vi "Add Tx UDP Section and Status Channels.vi"(8 "error in":errorcluster, 10 "Tx UDP configuration":T7(array[cluster]) {"sapPorts"."Parameters"."Parameter"."encoding" items=["BNR", "BCD", "Discrete"]; "commPorts"."Parameters"."Parameter"."encoding" items=["BNR", "BCD", "Discrete"]; "tx_udp_setup"."NumOfSubVl" format="%.0b"; "tx_udp_setup"."NetSelect" items=["FDX_TX_FRAME_DLY_A", "FDX_TX_FRAME_DLY_B", "FDX_TX_FRAME_BOTH", "FDX_TX_FRAME_ONLY_A", "FDX_TX_FRAME_ONLY_B"]}, 11 "port ref":T8 format="%.0x") -> (0 "error out":errorcluster, 3 "port ref out":T8 format="%.0x")   [LabVIEW 2020, in "AIM ARINC 664 Scripting.lvlib"]
doc: "Add a TX UDP page and status pages based on the Tx UDP configuration."
uses:
  AIM ARINC 664 Scripting.lvlib
  <vilib>/NI VeriStand/Custom Device API/Custom Device Item Ref.ctl
  <vilib>/NI VeriStand/Custom Device API/Custom Device API.lvlib
  Import/_typedefs/frame_parameter_definition.ctl
  Import/AIM ARINC 664 Import.lvlib
  Import/_typedefs/tx_udp_setup.ctl
  Import/_typedefs/frame_parameter.ctl
  Import/_typedefs/port_tx_udp_comm.ctl
  Import/_typedefs/port_tx_udp_sap.ctl
  Shared/Encoding (Arinc664).ctl
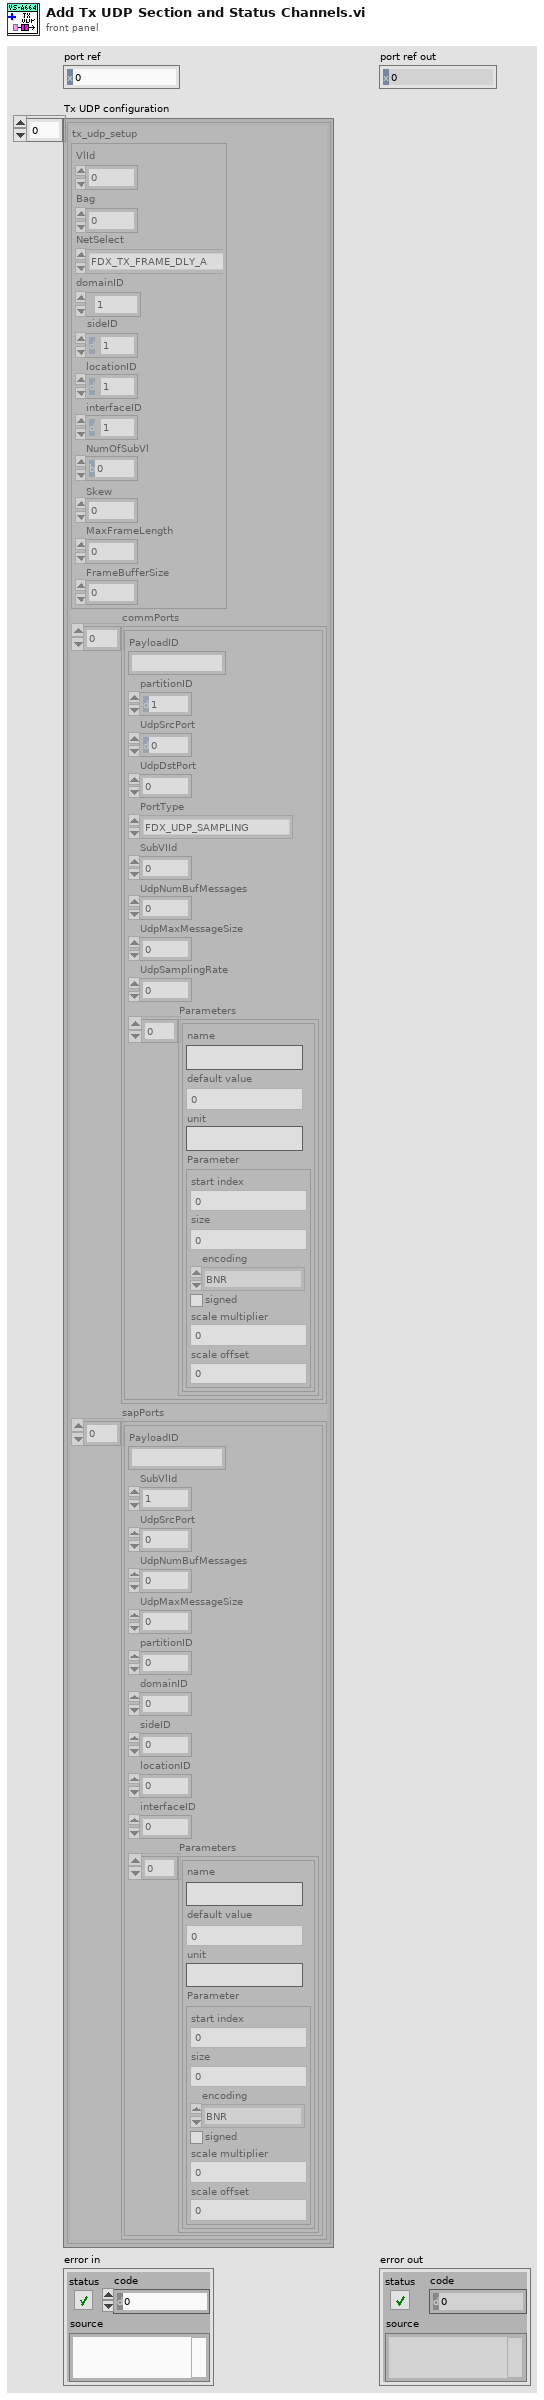
[diagram p1: front panel]
types:
  T1 = typedef "AIM ARINC 664 Import.lvlib/tx_udp_setup.ctl" = cluster{"VlId":i32, "Bag":i32, "NetSelect":u32, "domainID":u8, "sideID":u8, "locationID":u8, "interfaceID":u8, "NumOfSubVl":u16, "Skew":u32, "MaxFrameLength":u32, "FrameBufferSize":u32}
  T2 = typedef "AIM ARINC 664 Import.lvlib/port_tx_udp_comm.ctl" = cluster{"PayloadID":string, "partitionID":u8, "UdpSrcPort":u16, "UdpDstPort":u16, "PortType":enum16{"FDX_UDP_SAMPLING", "FDX_UDP_QUEUING"}, "SubVIId":u32, "UdpNumBufMessages":u32, "UdpMaxMessageSize":u32, "UdpSamplingRate":u32, "Parameters":T3[]}
  T3 = typedef "AIM ARINC 664 Import.lvlib/frame_parameter.ctl" = cluster{"name":string, "default value":dbl, "unit":string, "Parameter":T4}
  T4 = typedef "AIM ARINC 664 Import.lvlib/frame_parameter_definition.ctl" = cluster{"start index":i32, "size":i32, "encoding":T5, "signed":bool, "scale multiplier":dbl, "scale offset":dbl}
  T5 = typedef "Encoding (Arinc664).ctl" = u16
  T6 = typedef "AIM ARINC 664 Import.lvlib/port_tx_udp_sap.ctl" = cluster{"PayloadID":string, "SubVlId":u8, "UdpSrcPort":u16, "UdpNumBufMessages":u32, "UdpMaxMessageSize":u32, "partitionID":u8, "domainID":u8, "sideID":u8, "locationID":u8, "interfaceID":u8, "Parameters":T3[]}
  T7 = cluster{"tx_udp_setup":T1, "commPorts":T2[], "sapPorts":T6[]}[]
  T8 = typedef "Custom Device API.lvlib/Custom Device Item Ref.ctl" = u64
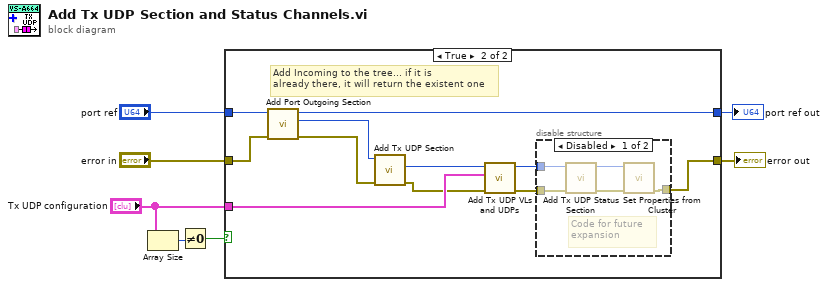
[diagram p0: block diagram]
diagram:
  n1 = Array Size(array="Tx UDP configuration") -> (size(s)=w3:i32)
  n2 = Not Equal To 0?(x=w3) -> (x != 0?=w2:bool)
  n3 = case shown="True" w2 {
    tunnel: [w8 w20] -> w7
    tunnel: "error in" -> [w8 w19]
    tunnel: "port ref" -> [w9 w18]
    tunnel: [w9 w15] -> w4
    tunnel: "Tx UDP configuration" -> [_ w14]
    frame False {
      # "If Tx_Udp Cluster is empty, bypass this"
    }
    frame True {
      # "Add Incoming to the tree... if it is \nalready there, it will return the existent one"
      n4 = call "Add Port Outgoing Section.vi"("error in"=w19, "ports ref"=w18) -> ("error out"=w17:errorcluster, "port outgoing ref out"=w16:T8, "ports ref out"=w15:T8)  [unwired: 7 in]
      n5 = call "Add Tx UDP Section.vi"("error in"=w17, "port outgoing ref"=w16) -> ("error out"=w12:errorcluster, "Tx UDP ref out"=w13:T8)  [unwired: 7 in, 1 out]
      n6 = call "Add Tx UDP VLs and UDPs.vi"("error in"=w12, "Tx UDP configuration"=w14, "Tx UDP ref"=w13) -> ("error out"=w11:errorcluster, "Tx UDP ref out"=w10:T8)  [unwired: 7 in]
      n7 = disable-structure shown="Disabled" {
        disable-tunnel: [w25 w26] -> w20
        disable-tunnel: w11 -> [w23 w26]
        disable-tunnel: w10 -> [w24 _]
        frame Disabled {
          # "Code for future \nexpansion"
          n8 = call "Add Tx UDP Status Section.vi"("error in"=w23, "Tx UDP ref"=w24) -> ("error out"=w21:errorcluster, "Tx UDP ref out"=w22:T8)  [unwired: 6 in, 2 out]
          n9 = call "Set Properties from Cluster.vi"("error in"=w21, "item ref in"=w22) -> ("error out"=w25:errorcluster)  [unwired: 8 in, 1 out]
        }
        frame Enabled {
        }
      }
    }
  }
  "error out" <- w7
  "port ref out" <- w4
